vi "Analyser.vi"() -> ()   [LabVIEW 2016]
panel:
  in  "Sair":bool
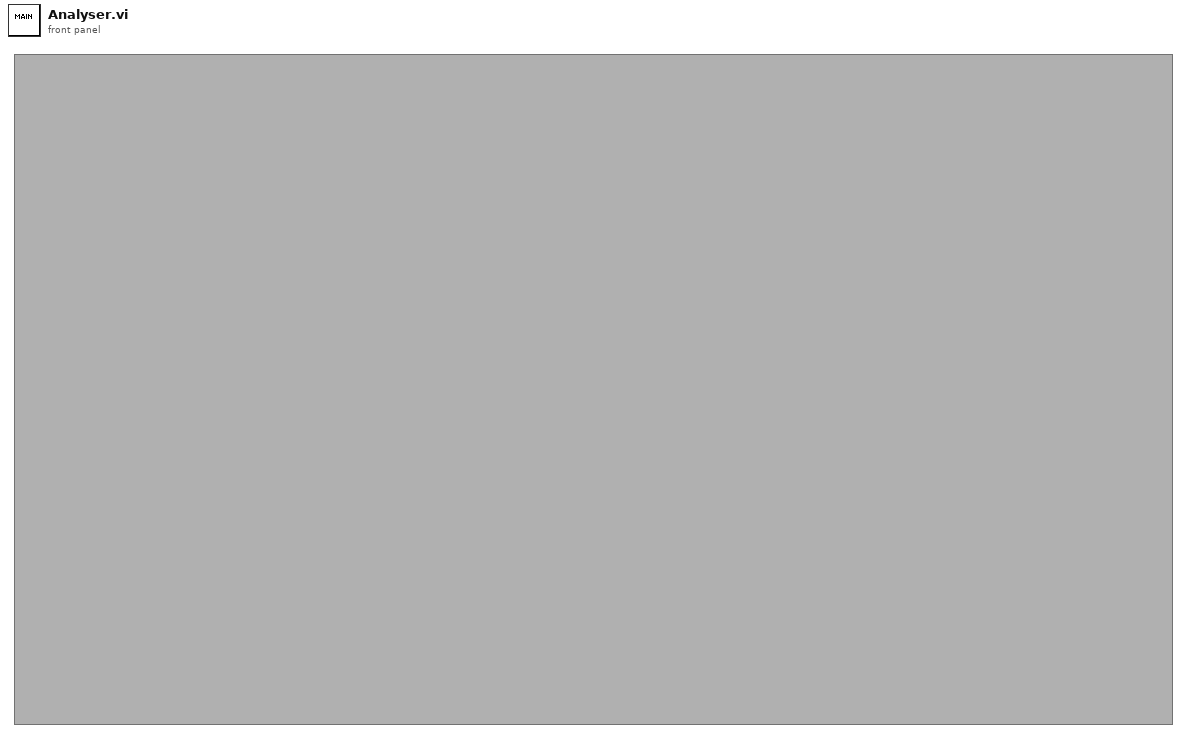
[diagram p1: front panel]
types:
  T1 = enum16{"Always On", "Always Off", "Off While Running"}
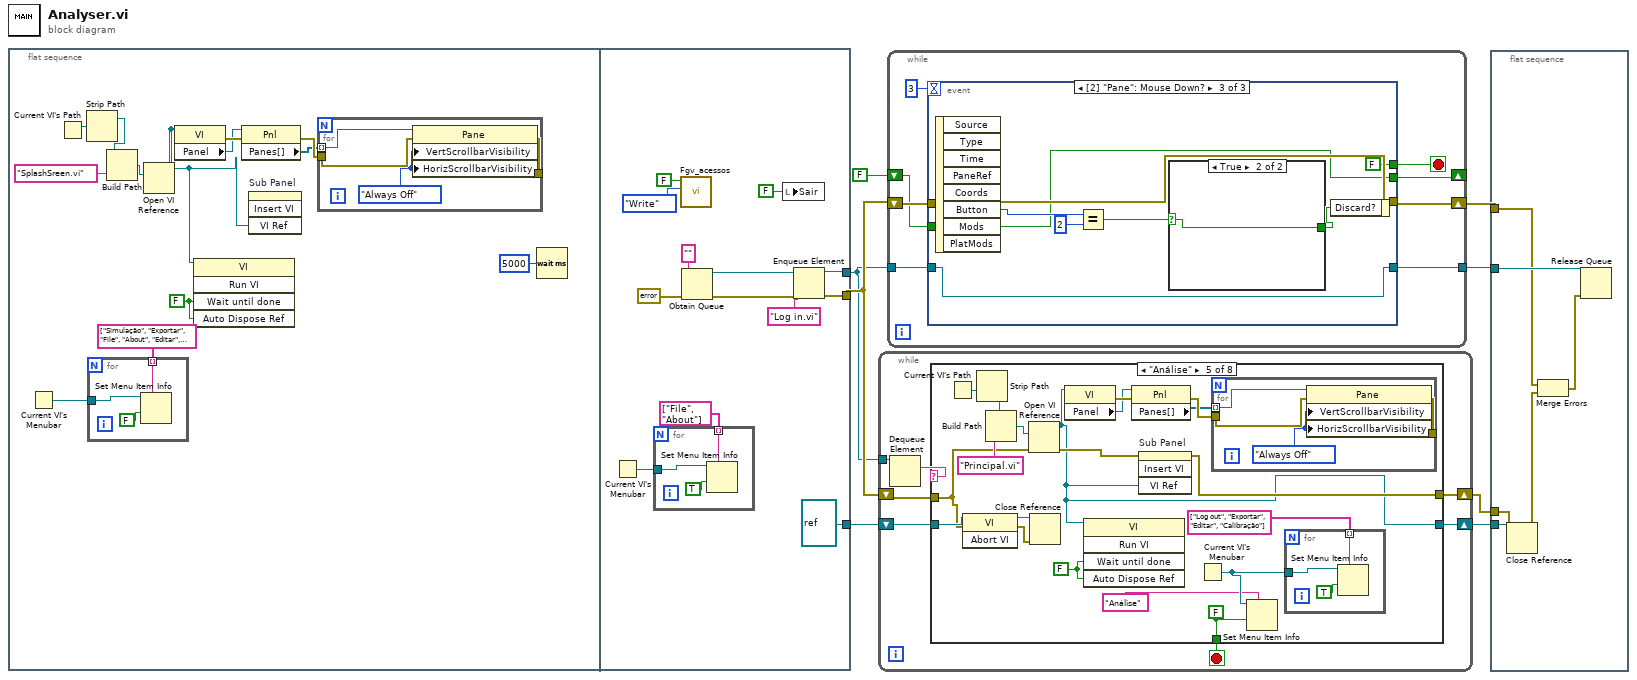
[diagram p0: block diagram]
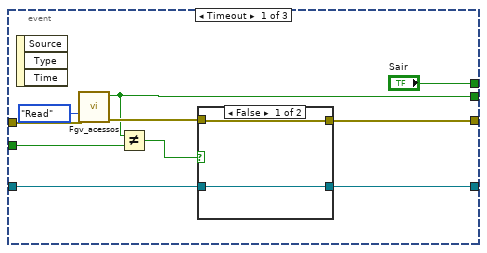
[diagram p2: hidden frame]
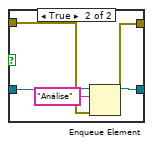
[diagram p3: hidden frame]
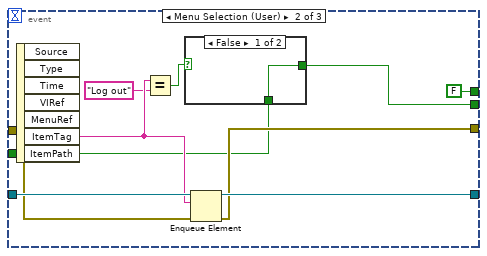
[diagram p4: hidden frame]
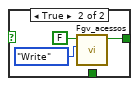
[diagram p5: hidden frame]
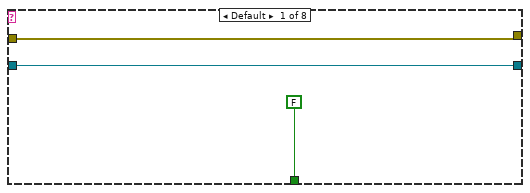
[diagram p7: hidden frame]
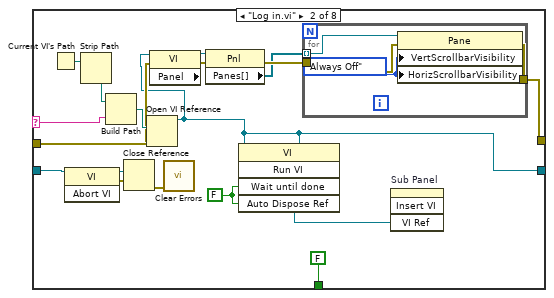
[diagram p8: hidden frame]
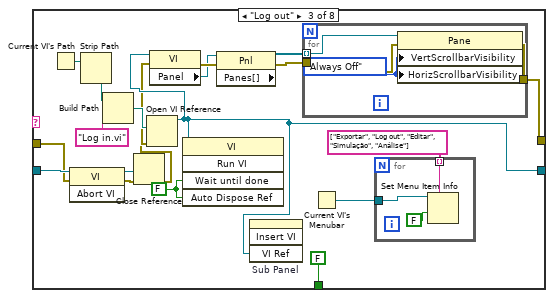
[diagram p9: hidden frame]
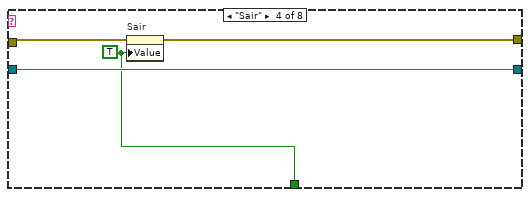
[diagram p10: hidden frame]
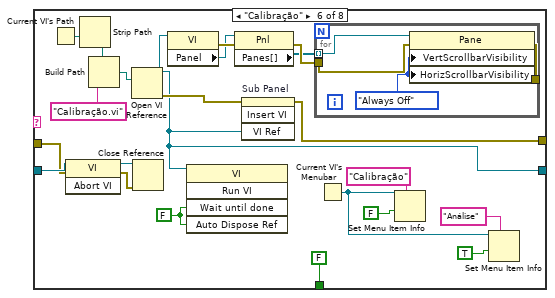
[diagram p11: hidden frame]
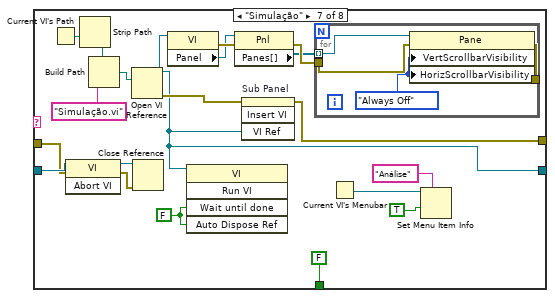
[diagram p12: hidden frame]
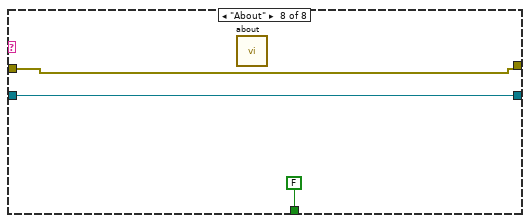
[diagram p13: hidden frame]
diagram:
  n1 = flat-sequence {
    tunnel: [w29] -> w1
    tunnel: [w37] -> w5
    tunnel: [refnum<vi> refnum ("vi reference")] -> w2
    frame #0 {
      w18 = FALSE ("Wait Until Done")
      n2 = Current VI's Menubar() -> (w10:refnum<k9>)
      n3 = Current VI's Path() -> (path=w12:path)
      n4 = Strip Path(path=w12) -> (stripped path=w13:path)  [unwired: 1 out]
      n5 = for {
        tunnel: w10 -> [w23]
        tunnel: string[] ["Simulação", "Exportar", "File", "About", "Editar", "Log out", "Análise"] -> [w22] mode=indexing
        n6 = Set Menu Item Info(7:w22, 9:FALSE ("enabled"), 11:w23) -> ()  [unwired: 4 in, 2 out]
      }
      n7 = Build Path(base path=w13, name or relative path="SplashSreen.vi") -> (appended path=w14:path)
      n8 = Open VI Reference(vi path=w14) -> (vi reference=w17:refnum<vi>)  [unwired: 5 in, 1 out]
      n9 = property class="VI"(reference=w17) -> (error out=w20:errorcluster, "Panel"=w15:refnum<vi>)  [unwired: 1 in, 1 out]
      n10 = invoke class="VI" method="Run VI"(reference=w17, "Wait until done"=w18, "Auto Dispose Ref"=w18) -> ()  [unwired: 2 in, 5 out]
      n11 = property class="Pnl"(reference=w15, error in=w20) -> (error out=w19:errorcluster, "Panes[]"=w16:refnum<vi>[])  [unwired: 1 out]
      n12 = invoke on="Sub Panel" class="SubPnl" method="Insert VI"("VI Ref"=w17) -> ()  [unwired: 3 in, 4 out]
      n13 = for {
        tunnel: w19 -> [w28]
        tunnel: [w27] -> _
        tunnel: w16 -> [w26] mode=indexing
        w25 = T1."Always Off" ("Vertical Scrollbar Visibility")
        n14 = property class="Pane"(reference=w26, error in=w28, "VertScrollbarVisibility"=w25, "HorizScrollbarVisibility"=w25) -> (error out=w27:errorcluster)  [unwired: 1 out]
      }
      n15 = Wait (ms)(milliseconds to wait=u32 5000) -> ()  [unwired: 1 out]
    }
    frame #1 {
      n16 = Current VI's Menubar() -> (w31:refnum<k9>)
      n17 = for {
        tunnel: w31 -> [w43]
        tunnel: string[] ["File", "About"] -> [w42] mode=indexing
        n18 = Set Menu Item Info(7:w42, 9:TRUE ("enabled"), 11:w43) -> ()  [unwired: 4 in, 2 out]
      }
      n19 = call "Fgv_acessos.vi"("Tipo"=enum16{"Write", "Read"}."Write", "Log in _acesso"=FALSE) -> ()  [unwired: 8 in, 2 out]
      n20 = Obtain Queue(element data type="", error in (no error)=errorcluster {"status"=FALSE, "code"=0, "source"=""} ("error constant")) -> (queue out=w40:refnum<queue>, error out=w38:errorcluster)  [unwired: 3 in, 1 out]
      n21 = local write "Sair"(FALSE ("Sair")) -> ()
      n22 = Enqueue Element(queue=w40, element="Log in.vi", error in (no error)=w38) -> (queue out=w29:refnum<queue>, error out=w37:errorcluster)  [unwired: 1 in, 1 out]
    }
  }
  n23 = while {
    tunnel: w1 -> [w51]
    shift-right: [w47] -> w6
    shift-left: w5 -> [w49]
    shift-right: [w46] -> w4
    shift-left: w2 -> [w45]
    stop <- w48 stop-if-true
    n24 = Dequeue Element(queue=w51) -> (element=w50:string)  [unwired: 2 in, 3 out]
    n25 = case shown="\"Análise\"" w50 {
      selector: w50 -> [_ w63 _ _ _ _ _ _]
      tunnel: w49 -> [w54 w72 w79 w105 w110 w135 w165 w187]
      tunnel: [FALSE ("Value") FALSE ("Value") FALSE ("Value") w106 w111 FALSE ("Value") FALSE ("Value") FALSE ("Value")] -> w48
      tunnel: [w54 w67 w92 w104 w125 w154 w178 w187] -> w47
      tunnel: [w52 w59 w90 w107 w114 w142 w164 w186] -> w46
      tunnel: w45 -> [w52 w58 w83 w107 w117 w145 w169 w186]
      frame Default {
      }
      frame "Log in.vi" {
        w71 = FALSE
        n26 = Current VI's Path() -> (path=w61:path)
        n27 = invoke class="VI" method="Abort VI"(reference=w58) -> (reference out=w56:refnum<vi>, error out=w57:errorcluster)  [unwired: 2 in, 1 out]
        n28 = Strip Path(path=w61) -> (stripped path=w60:path)  [unwired: 1 out]
        n29 = Build Path(base path=w60, name or relative path=w63) -> (appended path=w65:path)
        n30 = Close Reference(reference=w56, error in (no error)=w57) -> (error out=w55:errorcluster)
        n31 = Open VI Reference(vi path=w65, error in (no error)=w72) -> (vi reference=w59:refnum<vi>, error out=w64:errorcluster)  [unwired: 4 in]
        n32 = property class="VI"(reference=w59, error in=w64) -> (error out=w70:errorcluster, "Panel"=w69:refnum<vi>)  [unwired: 1 out]
        n33 = call <vilib>:"Clear Errors.vi"("error in (no error)"=w55) -> ()  [unwired: 5 in, 2 out]
        n34 = property class="Pnl"(reference=w69, error in=w70) -> (error out=w68:errorcluster, "Panes[]"=w62:refnum<vi>[])  [unwired: 1 out]
        n35 = invoke class="VI" method="Run VI"(reference=w59, "Wait until done"=w71, "Auto Dispose Ref"=w71) -> ()  [unwired: 2 in, 5 out]
        n36 = for {
          tunnel: w68 -> [w76]
          tunnel: [w75] -> w67
          tunnel: w62 -> [w74] mode=indexing
          w73 = T1."Always Off" ("Vertical Scrollbar Visibility")
          n37 = property class="Pane"(reference=w74, error in=w76, "VertScrollbarVisibility"=w73, "HorizScrollbarVisibility"=w73) -> (error out=w75:errorcluster)  [unwired: 1 out]
        }
        n38 = invoke on="Sub Panel" class="SubPnl" method="Insert VI"("VI Ref"=w59) -> ()  [unwired: 3 in, 4 out]
      }
      frame "Log out" {
        w96 = FALSE
        n39 = Current VI's Path() -> (path=w86:path)
        n40 = invoke class="VI" method="Abort VI"(reference=w83, error in=w79) -> (reference out=w81:refnum<vi>, error out=w80:errorcluster)  [unwired: 1 in, 1 out]
        n41 = Strip Path(path=w86) -> (stripped path=w85:path)  [unwired: 1 out]
        n42 = Build Path(base path=w85, name or relative path="Log in.vi" ("element")) -> (appended path=w89:path)
        n43 = Close Reference(reference=w81, error in (no error)=w80) -> (error out=w78:errorcluster)
        n44 = Open VI Reference(vi path=w89, error in (no error)=w78) -> (vi reference=w90:refnum<vi>, error out=w88:errorcluster)  [unwired: 4 in]
        n45 = property class="VI"(reference=w90, error in=w88) -> (error out=w95:errorcluster, "Panel"=w94:refnum<vi>)  [unwired: 1 out]
        n46 = invoke class="VI" method="Run VI"(reference=w90, "Wait until done"=w96, "Auto Dispose Ref"=w96) -> ()  [unwired: 2 in, 5 out]
        n47 = property class="Pnl"(reference=w94, error in=w95) -> (error out=w93:errorcluster, "Panes[]"=w87:refnum<vi>[])  [unwired: 1 out]
        n48 = invoke on="Sub Panel" class="SubPnl" method="Insert VI"("VI Ref"=w90) -> ()  [unwired: 3 in, 4 out]
        n49 = for {
          tunnel: w93 -> [w103]
          tunnel: [w102] -> w92
          tunnel: w87 -> [w101] mode=indexing
          w100 = T1."Always Off" ("Vertical Scrollbar Visibility")
          n50 = property class="Pane"(reference=w101, error in=w103, "VertScrollbarVisibility"=w100, "HorizScrollbarVisibility"=w100) -> (error out=w102:errorcluster)  [unwired: 1 out]
        }
        n51 = Current VI's Menubar() -> (w82:refnum<k9>)
        n52 = for {
          tunnel: w82 -> [w98]
          tunnel: string[] ["Exportar", "Log out", "Editar", "Simulação", "Análise"] -> [w97] mode=indexing
          n53 = Set Menu Item Info(7:w97, 9:FALSE ("enabled"), 11:w98) -> ()  [unwired: 4 in, 2 out]
        }
      }
      frame "Sair" {
        w106 = TRUE ("Sair")
        n54 = property on="Sair" class="Bool (strict)"(error in=w105, "Value"=w106) -> (error out=w104:errorcluster)  [unwired: 1 in, 1 out]
      }
      frame "Análise" {
        w111 = FALSE ("Value")
        w118 = FALSE
        n55 = Current VI's Path() -> (path=w124:path)
        n56 = invoke class="VI" method="Abort VI"(reference=w117, error in=w110) -> (reference out=w116:refnum<vi>, error out=w115:errorcluster)  [unwired: 1 in, 1 out]
        n57 = Strip Path(path=w124) -> (stripped path=w123:path)  [unwired: 1 out]
        n58 = Build Path(base path=w123, name or relative path="Principal.vi") -> (appended path=w127:path)
        n59 = Open VI Reference(vi path=w127, error in (no error)=w110) -> (vi reference=w114:refnum<vi>, error out=w126:errorcluster)  [unwired: 4 in]
        n60 = Close Reference(reference=w116, error in (no error)=w115) -> ()  [unwired: 1 out]
        n61 = property class="VI"(reference=w114) -> (error out=w122:errorcluster, "Panel"=w121:refnum<vi>)  [unwired: 1 in, 1 out]
        n62 = invoke class="VI" method="Run VI"(reference=w114, "Wait until done"=w118, "Auto Dispose Ref"=w118) -> ()  [unwired: 2 in, 5 out]
        n63 = property class="Pnl"(reference=w121, error in=w122) -> (error out=w120:errorcluster, "Panes[]"=w119:refnum<vi>[])  [unwired: 1 out]
        n64 = invoke on="Sub Panel" class="SubPnl" method="Insert VI"(error in=w126, "VI Ref"=w114) -> (error out=w125:errorcluster)  [unwired: 2 in, 3 out]
        n65 = Current VI's Menubar() -> (w112:refnum<k9>)
        n66 = for {
          tunnel: w120 -> [w134]
          tunnel: [w133] -> _
          tunnel: w119 -> [w132] mode=indexing
          w131 = T1."Always Off" ("Vertical Scrollbar Visibility")
          n67 = property class="Pane"(reference=w132, error in=w134, "VertScrollbarVisibility"=w131, "HorizScrollbarVisibility"=w131) -> (error out=w133:errorcluster)  [unwired: 1 out]
        }
        n68 = Set Menu Item Info(7:"Análise" ("item name"), 9:w111, 11:w112) -> ()  [unwired: 4 in, 2 out]
        n69 = for {
          tunnel: w112 -> [w129]
          tunnel: string[] ["Log out", "Exportar", "Editar", "Calibração"] -> [w128] mode=indexing
          n70 = Set Menu Item Info(7:w128, 9:TRUE ("enabled"), 11:w129) -> ()  [unwired: 4 in, 2 out]
        }
      }
      frame "Calibração" {
        w146 = FALSE
        n71 = Current VI's Path() -> (path=w152:path)
        n72 = invoke class="VI" method="Abort VI"(reference=w145, error in=w135) -> (reference out=w144:refnum<vi>, error out=w143:errorcluster)  [unwired: 1 in, 1 out]
        n73 = Strip Path(path=w152) -> (stripped path=w151:path)  [unwired: 1 out]
        n74 = Build Path(base path=w151, name or relative path="Calibração.vi") -> (appended path=w156:path)
        n75 = Open VI Reference(vi path=w156) -> (vi reference=w142:refnum<vi>, error out=w155:errorcluster)  [unwired: 5 in]
        n76 = Close Reference(reference=w144, error in (no error)=w143) -> ()  [unwired: 1 out]
        n77 = property class="VI"(reference=w142) -> (error out=w150:errorcluster, "Panel"=w149:refnum<vi>)  [unwired: 1 in, 1 out]
        n78 = invoke class="VI" method="Run VI"(reference=w142, "Wait until done"=w146, "Auto Dispose Ref"=w146) -> ()  [unwired: 2 in, 5 out]
        n79 = property class="Pnl"(reference=w149, error in=w150) -> (error out=w148:errorcluster, "Panes[]"=w147:refnum<vi>[])  [unwired: 1 out]
        n80 = invoke on="Sub Panel" class="SubPnl" method="Insert VI"(error in=w155, "VI Ref"=w142) -> (error out=w154:errorcluster)  [unwired: 2 in, 3 out]
        n81 = for {
          tunnel: w148 -> [w160]
          tunnel: [w159] -> _
          tunnel: w147 -> [w158] mode=indexing
          w157 = T1."Always Off" ("Vertical Scrollbar Visibility")
          n82 = property class="Pane"(reference=w158, error in=w160, "VertScrollbarVisibility"=w157, "HorizScrollbarVisibility"=w157) -> (error out=w159:errorcluster)  [unwired: 1 out]
        }
        n83 = Current VI's Menubar() -> (w136:refnum<k9>)
        n84 = Set Menu Item Info(7:"Calibração", 9:FALSE ("enabled"), 11:w136) -> ()  [unwired: 4 in, 2 out]
        n85 = Set Menu Item Info(7:"Análise", 9:TRUE ("enabled"), 11:w136) -> ()  [unwired: 4 in, 2 out]
      }
      frame "Simulação" {
        w170 = FALSE
        n86 = Current VI's Path() -> (path=w176:path)
        n87 = invoke class="VI" method="Abort VI"(reference=w169, error in=w165) -> (reference out=w168:refnum<vi>, error out=w167:errorcluster)  [unwired: 1 in, 1 out]
        n88 = Strip Path(path=w176) -> (stripped path=w175:path)  [unwired: 1 out]
        n89 = Build Path(base path=w175, name or relative path="Simulação.vi") -> (appended path=w180:path)
        n90 = Open VI Reference(vi path=w180) -> (vi reference=w164:refnum<vi>, error out=w179:errorcluster)  [unwired: 5 in]
        n91 = Close Reference(reference=w168, error in (no error)=w167) -> ()  [unwired: 1 out]
        n92 = property class="VI"(reference=w164) -> (error out=w174:errorcluster, "Panel"=w173:refnum<vi>)  [unwired: 1 in, 1 out]
        n93 = invoke class="VI" method="Run VI"(reference=w164, "Wait until done"=w170, "Auto Dispose Ref"=w170) -> ()  [unwired: 2 in, 5 out]
        n94 = property class="Pnl"(reference=w173, error in=w174) -> (error out=w172:errorcluster, "Panes[]"=w171:refnum<vi>[])  [unwired: 1 out]
        n95 = invoke on="Sub Panel" class="SubPnl" method="Insert VI"(error in=w179, "VI Ref"=w164) -> (error out=w178:errorcluster)  [unwired: 2 in, 3 out]
        n96 = for {
          tunnel: w172 -> [w184]
          tunnel: [w183] -> _
          tunnel: w171 -> [w182] mode=indexing
          w181 = T1."Always Off" ("Vertical Scrollbar Visibility")
          n97 = property class="Pane"(reference=w182, error in=w184, "VertScrollbarVisibility"=w181, "HorizScrollbarVisibility"=w181) -> (error out=w183:errorcluster)  [unwired: 1 out]
        }
        n98 = Current VI's Menubar() -> (w161:refnum<k9>)
        n99 = Set Menu Item Info(7:"Análise", 9:TRUE ("enabled"), 11:w161) -> ()  [unwired: 4 in, 2 out]
      }
      frame "About" {
        n100 = call "about.vi"() -> ()  [unwired: 12 in]
      }
    }
  }
  n101 = while {
    shift-right: [w192] -> w8
    shift-left: w5 -> [w193]
    tunnel: w1 -> [w191]
    tunnel: [w190] -> w7
    shift-right: [w189] -> _
    shift-left: FALSE ("Acesso permitido") -> [w188]
    stop <- w194 stop-if-true
    n102 = event shown="[2] \"Pane\": Mouse Down?" {
      selector: _ -> [_ _ _]
      dyn-events: _ -> [_ _ _]
      timeout: 3 -> [_ _ _]
      tunnel: ["Sair" FALSE ("Sair") FALSE ("Sair")] -> w194
      tunnel: w193 -> [w203 w220 w229]
      tunnel: [w199 w219 w229] -> w192
      tunnel: w191 -> [w202 w222 w230]
      tunnel: [w201 w221 w230] -> w190
      tunnel: [w198 w214 w228] -> w189
      tunnel: w188 -> [w197 w213 w228]
      event Timeout {
        n103 = event-data() -> ()  [unwired: 1 in, 3 out]
        n104 = call "Fgv_acessos.vi"("error in"=w203, "Tipo"=enum16{"Write", "Read"}."Read") -> ("Error out"=w200:errorcluster, "Acesso permitido"=w198:bool)  [unwired: 8 in]
        n105 = Not Equal?(x=w198, y=w197) -> (x != y?=w196:bool)
        n106 = case shown="False" w196 {
          tunnel: w202 -> [w206 w212]
          tunnel: [w206 w211] -> w201
          tunnel: w200 -> [w207 w210]
          tunnel: [w207 w209] -> w199
          frame False {
          }
          frame True {
            n107 = Enqueue Element(queue=w212, element="Análise", error in (no error)=w210) -> (queue out=w211:refnum<queue>, error out=w209:errorcluster)  [unwired: 1 in, 1 out]
          }
        }
      }
      event Menu Selection (User) {
        n108 = event-data() -> ("ItemTag"=w218:string)  [unwired: 1 in, 6 out]
        n109 = Equal?(x=w218, y="Log out") -> (x = y?=w216:bool)
        n110 = case shown="False" w216 {
          tunnel: [w223 w224] -> w214
          tunnel: w213 -> [w223 _]
          frame False {
          }
          frame True {
            n111 = call "Fgv_acessos.vi"("Tipo"=enum16{"Write", "Read"}."Write", "Log in _acesso"=FALSE) -> ("Acesso permitido"=w224:bool)  [unwired: 8 in, 1 out]
          }
        }
        n112 = Enqueue Element(queue=w222, element=w218, error in (no error)=w220) -> (queue out=w221:refnum<queue>, error out=w219:errorcluster)  [unwired: 1 in, 1 out]
      }
      event Mouse Down? {
        n113 = event-data() -> ("Button"=w234:u16)  [unwired: 1 in, 7 out]
        n114 = Equal?(x=w234, y=u16 2) -> (x = y?=w232:bool)
        n115 = case shown="True" w232 {
          selector: w232 -> [w235 w236]
          tunnel: [w235 w236] -> w231
          frame False {
          }
          frame True {
          }
        }
        n116 = event-data("Discard?"=w231) -> ()  [unwired: 1 in, 1 out]
      }
    }
  }
  n117 = flat-sequence {
    tunnel: w8 -> [w241]
    tunnel: w7 -> [w242]
    tunnel: w6 -> [w238]
    tunnel: w4 -> [w239]
    frame #0 {
      n118 = Close Reference(reference=w239, error in (no error)=w238) -> (error out=w237:errorcluster)
      n119 = Merge Errors(w241, w237) -> (w240:errorcluster)
      n120 = Release Queue(queue=w242, error in (no error)=w240) -> ()  [unwired: 1 in, 3 out]
    }
  }
